vi "readFromXML.vi"(8 "error in (no error)":errorcluster, 10 "XML in":string="<RADecTarget>\n  <parallax_Arcsec>1.111</parallax_Arcsec>\n  <properMotion>\n    <epochPM_Yr>2010</epochPM_Yr>\n    <pmdec_ArcsPYr>1.111</pmdec_ArcsPYr>\n    <pmra_SPYr>2.222</pmra_SPYr>\n  </properMotion>\n  <rv_kps>3.333</rv_kps>\n  <targetName>ThisIsIt</targetName>\n  <DifftrackRADec>\n    <dDec_ArcsPS>1</dDec_ArcsPS>\n    <dRA_sps>112.2</dRA_sps>\n  </DifftrackRADec>\n</RADecTarget>", 11 "Target in":refnum<class "Target.lvclass">) -> (0 "error out":errorcluster, 3 "Target out":refnum<class "Target.lvclass">)   [LabVIEW 2014, in "TCSDataDefinitions.lvlib" / "TCSCommand.lvlib" / "TargetConfiguration.lvlib" / "Target.lvlib" / "Target.lvclass"]
uses:
  Target/Target.lvclass
  Target/Target.lvclass/Target.ctl
  Difftrack/Difftrack.lvclass
  <userlib>/Common/XML/XMLParser/XMLParser.lvclass
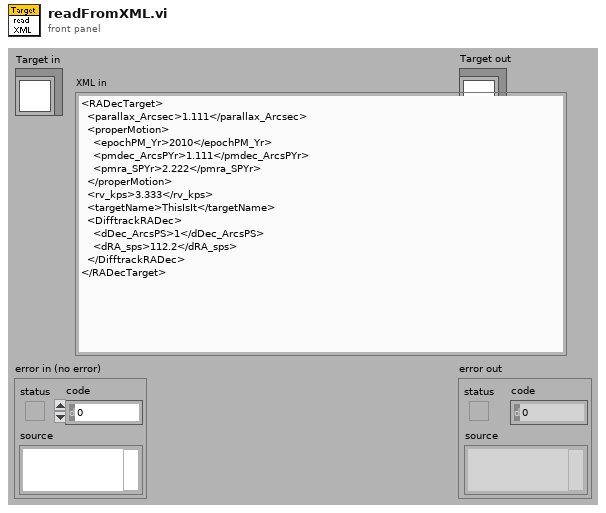
[diagram p1: front panel]
types:
  T1 = typedef "XML.lvlib/AttributeElements.ctl" = cluster{"attributeType":string, "attributeValue":string}
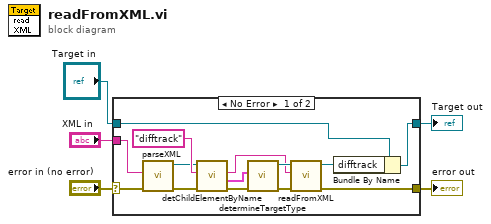
[diagram p0: block diagram]
diagram:
  n1 = case shown="No Error" "error in (no error)" {
    selector: "error in (no error)" -> [w18 w21]
    tunnel: [w13 w21] -> w4
    tunnel: [w15 w20] -> w2
    tunnel: "Target in" -> [w17 w20]
    tunnel: "XML in" -> [w19 _]
    frame No Error {
      n2 = call <userlib>:"parseXML.vi"("error in (no error)"=w18, "XMLString in"=w19) -> ("error out"=w12:errorcluster, "Element out"=w8:refnum<class "XMLParser.lvclass">)  [unwired: 8 in]
      n3 = call <userlib>:"detChildElementByName.vi"("error in (no error)"=w12, "childName"="difftrack" ("ChildName"), "Element in"=w8) -> ("error out"=w11:errorcluster, "childAttributes"=w6:T1[], "childXML"=w7:string)  [unwired: 5 in, 1 out]
      n4 = call "determineTargetType.vi"("error in (no error)"=w11, "childAttributes"=w6) -> ("error out"=w9:errorcluster, "Difftrack.lvclass"=w10:refnum<class "Difftrack.lvclass">)  [unwired: 8 in]
      n5 = call-dynamic "readFromXML.vi"("error in (no error)"=w9, "XML in"=w7, "Difftrack in"=w10) -> ("error out"=w13:errorcluster, "Difftrack out"=w14:refnum<class "Difftrack.lvclass">)  [unwired: 7 in]
      n6 = Bundle By Name(cluster=w17, "difftrack"=w14) -> (w15:refnum<class "Target.lvclass">)
    }
    frame Error {
    }
  }
  "error out" <- w4
  "Target out" <- w2
